vi "Adapt To Type.vi"(7 "Type and Defaults":variant, 8 "error in (no error)":errorcluster, 10 "Variant in":variant, 11 "Deserializer in":refnum<class "JSON Deserializer.lvclass">) -> (0 "error out":errorcluster, 2 "Variant out":variant, 3 "Deserializer out":refnum<class "JSON Deserializer.lvclass">)   [LabVIEW 2017, in "JKI JSON Serialization.lvlib" / "JSON Deserializer.lvclass"]
doc: "Adapts <b>Variant in</b> previously unflattened from a JSON formatted string to match the type of <b>Type and Defaults</b>. For any cluster element in Type and Defaults, the value of the element in Type and Default is used if element with the same name is not present in Variant in."
uses:
  JSON Deserializer.lvclass
  JSON Deserializer.lvclass/JSON Deserializer.ctl
  Library/Waveform Cluster.ctl
  Library/Empty Cluster.vi
  Library/Null Value.vi
  <vilib>/Utility/VariantDataType/VariantType.lvlib
  JKI JSON Serialization.lvlib
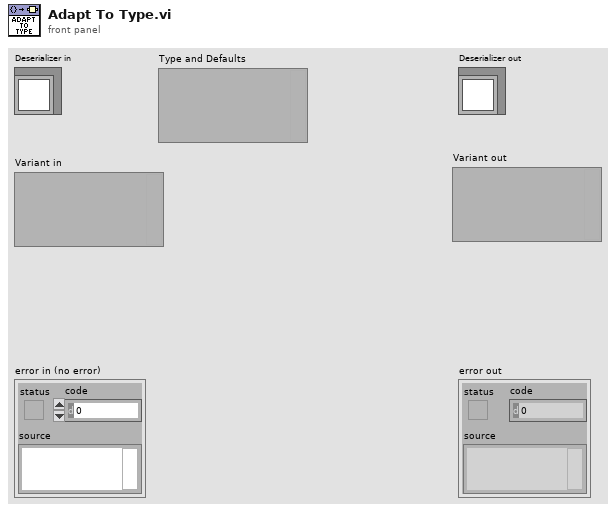
[diagram p1: front panel]
types:
  T1 = typedef "VariantType.lvlib/Type.ctl" = enum8{"Invalid Type", "Void", "I8", "I16", "I32", "I64", "U8", "U16", "U32", "U64", "Single Float", "Double Float", "Extended Float", "Single Complex", "Double Complex", "Extended Complex", "Enum U8", "Enum U16", "Enum U32", "Enum U64", "Single Float With Unit", "Double Float With Unit", "Extended Float With Unit", "Single Complex with Unit", "Double Complex with Unit", "Extended Complex with Unit", "Boolean", "String", "Path", "Picture", "Tag", "Array", "Cluster", "Variant", "LV Variant", "Waveform", "Timestamp", "Digital Waveform", "Digital Data", "ExpressData", "Refnum", "External Data", "VI", "Poly VI", "LabVIEW Class Instance", "Fixed Point"}
  T2 = typedef "JKI JSON Serialization.lvlib/Waveform Cluster.ctl" = cluster{"t0":timestamp, "dt":dbl, "y":dbl[]}
  T3 = typedef "VariantType.lvlib/MemoryInfo.ctl" = cluster{"Type":T4, "Size":u32}
  T4 = typedef "VariantType.lvlib/MemoryType.ctl" = enum16{"Variable", "Fixed", "Bounded"}
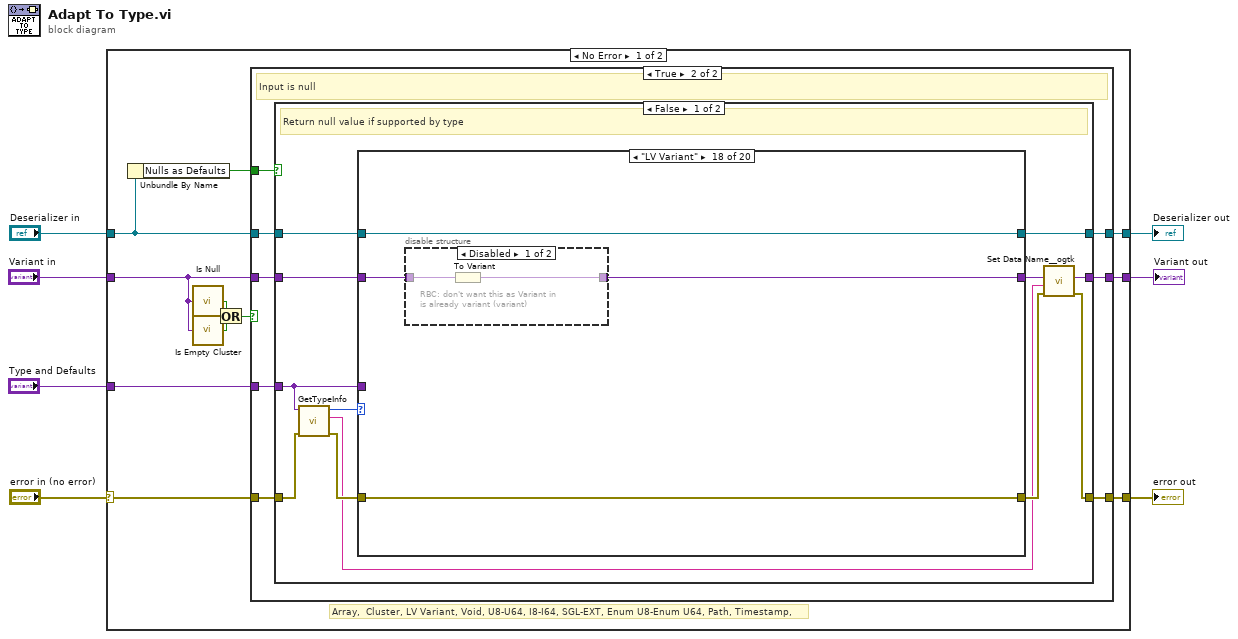
[diagram p0: block diagram]
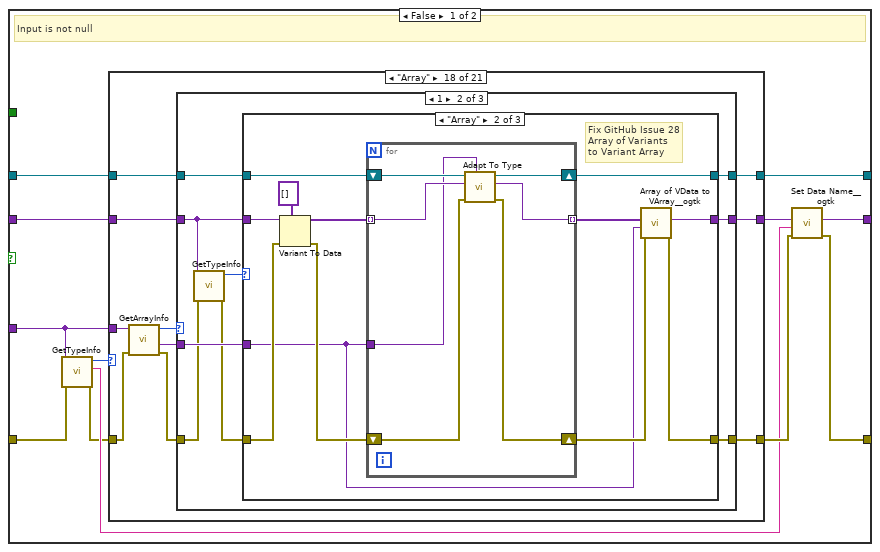
[diagram p2: hidden frame]
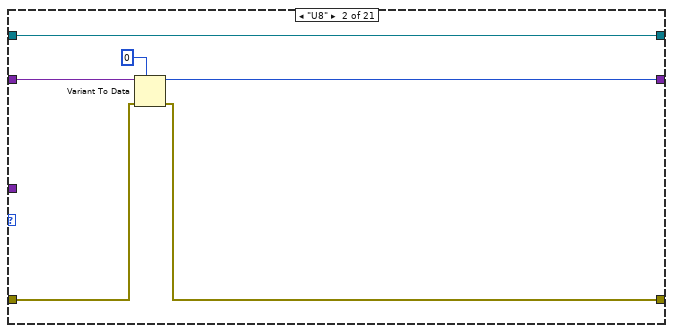
[diagram p4: hidden frame]
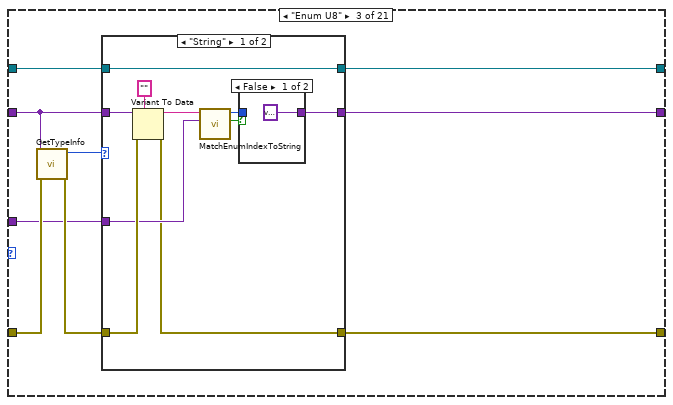
[diagram p5: hidden frame]
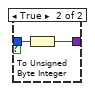
[diagram p6: hidden frame]
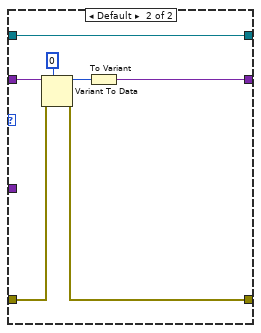
[diagram p7: hidden frame]
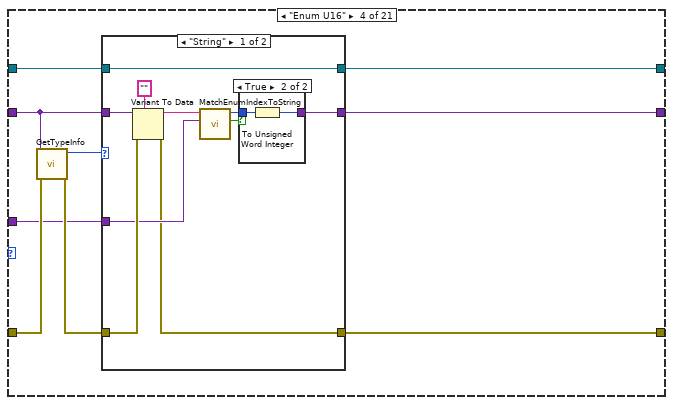
[diagram p8: hidden frame]
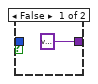
[diagram p9: hidden frame]
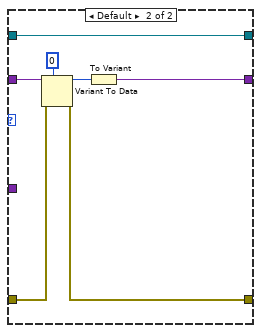
[diagram p10: hidden frame]
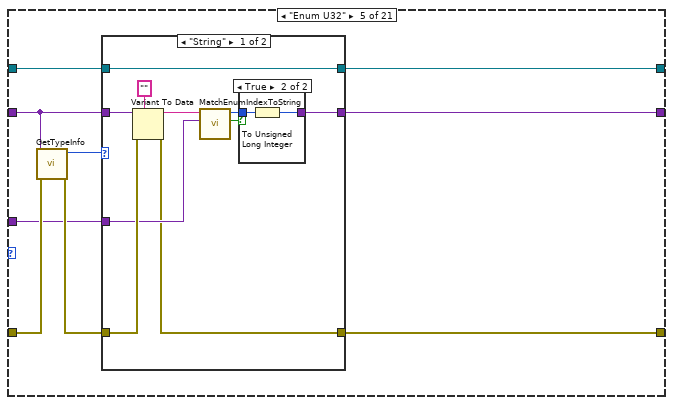
[diagram p11: hidden frame]
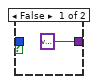
[diagram p12: hidden frame]
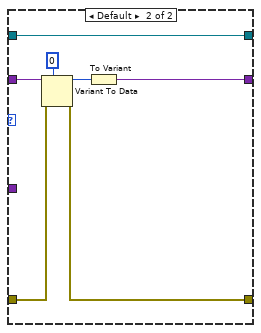
[diagram p13: hidden frame]
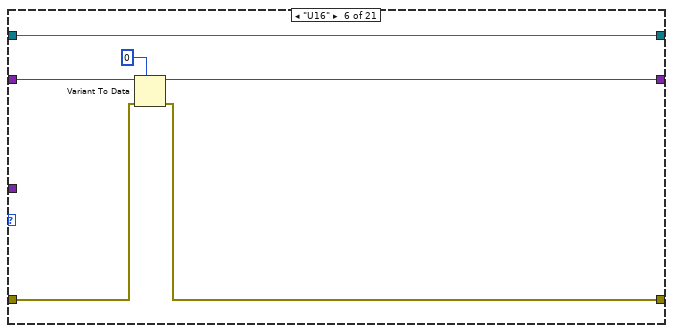
[diagram p14: hidden frame]
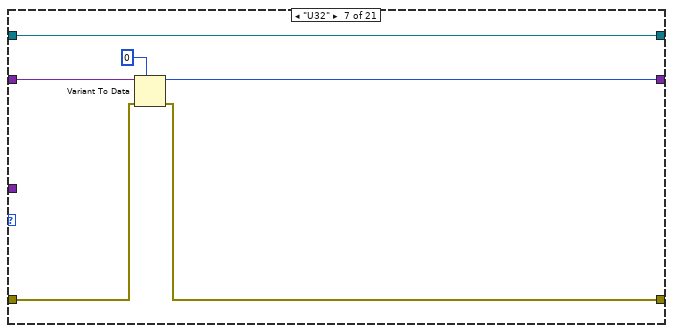
[diagram p15: hidden frame]
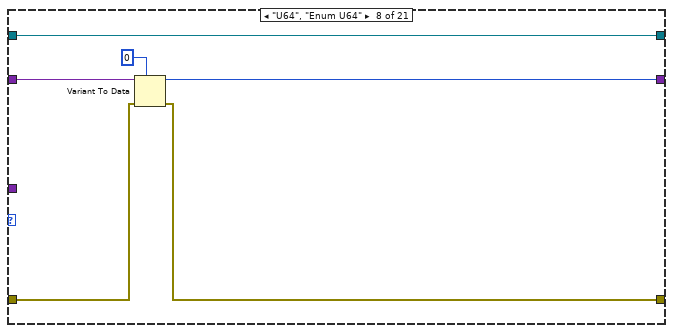
[diagram p16: hidden frame]
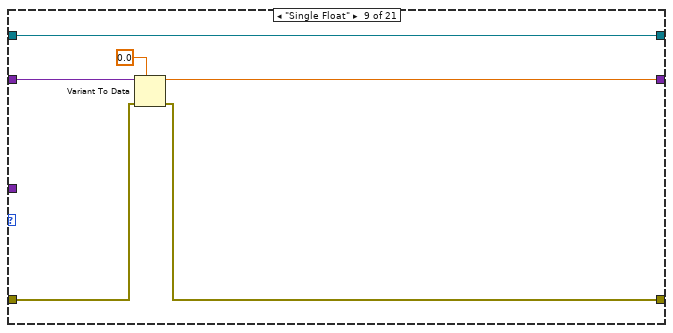
[diagram p17: hidden frame]
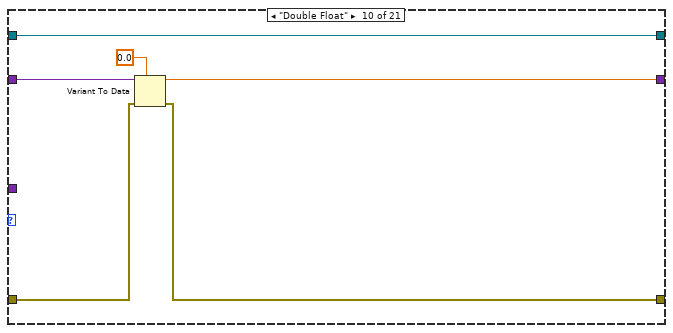
[diagram p18: hidden frame]
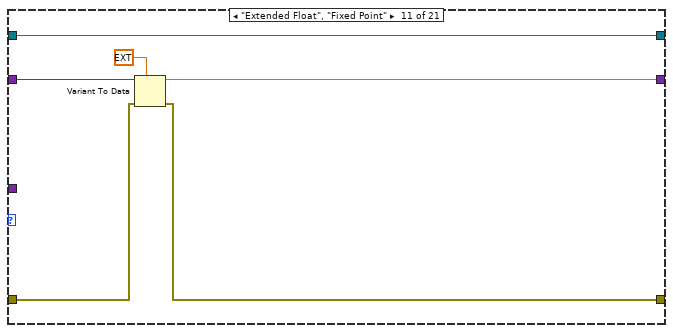
[diagram p19: hidden frame]
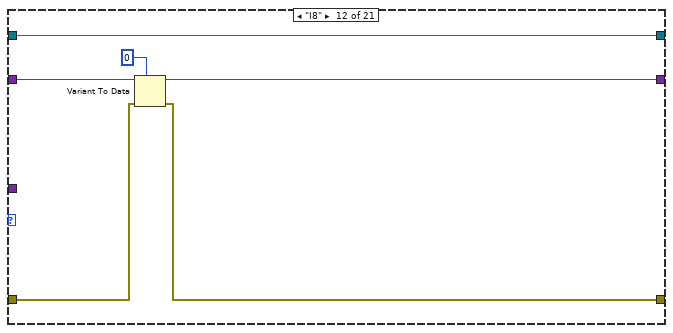
[diagram p20: hidden frame]
diagram:
  n1 = case shown="No Error" "error in (no error)" {
    selector: "error in (no error)" -> [w17 w553]
    tunnel: "Deserializer in" -> [w13 w554]
    tunnel: "Variant in" -> [w11 _]
    tunnel: [w14 w553] -> w4
    tunnel: "Type and Defaults" -> [w16 w552]
    tunnel: [w18 w554] -> w2
    tunnel: [w15 w552] -> w1
    frame No Error {
      # "Array,  Cluster, LV Variant, Void, U8-U64, I8-I64, SGL-EXT, Enum U8-Enum U64, Path, Timestamp,"
      n2 = Unbundle By Name(w13) -> ("Nulls as Defaults"=w12:bool)
      n3 = call "Is Null.vi"("Deserialized JSON Data"=w11) -> ("Null?"=w10:bool)
      n4 = call "Is Empty Cluster.vi"("Deserialized JSON Data"=w11) -> ("Empty Cluster?"=w9:bool)
      n5 = Or(x=w10, y=w9) -> (x .or. y?=w8:bool)
      n6 = case shown="True" w8 {
        tunnel: w13 -> [w20 w434]
        tunnel: [w19 w433] -> w18
        tunnel: w17 -> [w29 w431]
        tunnel: w16 -> [w28 w435]
        tunnel: [w26 w436] -> w15
        tunnel: [w25 w430] -> w14
        tunnel: w11 -> [w21 w432]
        tunnel: w12 -> [_ w429]
        frame False {
          # "Input is not null"
          n7 = call <vilib>:"GetTypeInfo.vi"("error in (no error)"=w29, "Variant"=w28) -> ("error out"=w22:errorcluster, "Name"=w23:string, "Type Enum"=w30:T1)  [unwired: 5 in, 2 out]
          n8 = case shown="\"Array\"" w30 {
            tunnel: [w32 w36 w46 w75 w104 w129 w135 w141 w147 w153 w159 w165 w171 w177 w183 w192 w195 w208 w293 w376 w426] -> w24
            tunnel: w22 -> [w32 w37 w44 w73 w102 w130 w136 w142 w148 w154 w160 w166 w172 w178 w184 w189 w199 w210 w292 w375 w426]
            tunnel: w20 -> [w33 w39 w42 w71 w100 w132 w138 w144 w150 w156 w162 w168 w174 w180 w186 w193 w201 w207 w297 w380 w428]
            tunnel: [w33 w39 w41 w70 w99 w132 w138 w144 w150 w156 w162 w168 w174 w180 w186 w193 w201 w205 w296 w379 w428] -> w19
            tunnel: w28 -> [_ _ w40 w69 w98 _ _ _ _ _ _ _ _ _ _ _ _ w211 w295 w378 _]
            tunnel: w21 -> [w31 w38 w47 w76 w105 w131 w137 w143 w149 w155 w161 w167 w173 w179 w185 w190 w200 w202 w290 w373 w427]
            tunnel: [w31 w34 w48 w77 w106 w127 w133 w139 w145 w151 w157 w163 w169 w175 w181 w191 w194 w204 w294 w377 w425] -> w27
            frame "Void", Default {
            }
            frame "U8" {
              n9 = Variant To Data(error in=w37, type=u8 0, Variant=w38) -> (data=w34:u8, error out=w36:errorcluster)
            }
            frame "Enum U8" {
              n10 = call <vilib>:"GetTypeInfo.vi"("error in (no error)"=w44, "Variant"=w47) -> ("error out"=w43:errorcluster, "Type Enum"=w45:T1)  [unwired: 5 in, 3 out]
              n11 = case shown="\"String\"" w45 {
                tunnel: [w52 w62] -> w48
                tunnel: w47 -> [w58 w66]
                tunnel: w43 -> [w56 w65]
                tunnel: [w49 w64] -> w46
                tunnel: w42 -> [w50 w63]
                tunnel: [w50 w63] -> w41
                tunnel: w40 -> [w54 _]
                frame "String" {
                  n12 = Variant To Data(error in=w56, type="", Variant=w58) -> (data=w55:string, error out=w49:errorcluster)
                  n13 = call "MatchEnumIndexToString.vi"("Enum Variant"=w54, "String"=w55) -> ("found"=w51:bool, "index"=w53:i32)  [unwired: 8 in]
                  n14 = case shown="False" w51 {
                    tunnel: w53 -> [_ w61]
                    tunnel: [variant ("Type and Defaults") w60] -> w52
                    frame False {
                    }
                    frame True {
                      n15 = To Unsigned Byte Integer(number=w61) -> (unsigned 8bit integer=w60:u8)
                    }
                  }
                }
                frame Default {
                  n16 = Variant To Data(error in=w65, type=u8 0, Variant=w66) -> (data=w67:u8, error out=w64:errorcluster)
                  n17 = To Variant(anything=w67) -> (Variant=w62:variant)
                }
              }
            }
            frame "Enum U16" {
              n18 = call <vilib>:"GetTypeInfo.vi"("error in (no error)"=w73, "Variant"=w76) -> ("error out"=w72:errorcluster, "Type Enum"=w74:T1)  [unwired: 5 in, 3 out]
              n19 = case shown="\"String\"" w74 {
                tunnel: [w81 w91] -> w77
                tunnel: w76 -> [w87 w95]
                tunnel: w72 -> [w85 w94]
                tunnel: [w78 w93] -> w75
                tunnel: w71 -> [w79 w92]
                tunnel: [w79 w92] -> w70
                tunnel: w69 -> [w83 _]
                frame "String" {
                  n20 = Variant To Data(error in=w85, type="", Variant=w87) -> (data=w84:string, error out=w78:errorcluster)
                  n21 = call "MatchEnumIndexToString.vi"("Enum Variant"=w83, "String"=w84) -> ("found"=w80:bool, "index"=w82:i32)  [unwired: 8 in]
                  n22 = case shown="True" w80 {
                    tunnel: w82 -> [_ w90]
                    tunnel: [variant ("Type and Defaults") w89] -> w81
                    frame False {
                    }
                    frame True {
                      n23 = To Unsigned Word Integer(number=w90) -> (unsigned 16bit integer=w89:u16)
                    }
                  }
                }
                frame Default {
                  n24 = Variant To Data(error in=w94, type=u16 0, Variant=w95) -> (data=w96:u16, error out=w93:errorcluster)
                  n25 = To Variant(anything=w96) -> (Variant=w91:variant)
                }
              }
            }
            frame "Enum U32" {
              n26 = call <vilib>:"GetTypeInfo.vi"("error in (no error)"=w102, "Variant"=w105) -> ("error out"=w101:errorcluster, "Type Enum"=w103:T1)  [unwired: 5 in, 3 out]
              n27 = case shown="\"String\"" w103 {
                tunnel: [w110 w120] -> w106
                tunnel: w105 -> [w116 w124]
                tunnel: w101 -> [w114 w123]
                tunnel: [w107 w122] -> w104
                tunnel: w100 -> [w108 w121]
                tunnel: [w108 w121] -> w99
                tunnel: w98 -> [w112 _]
                frame "String" {
                  n28 = Variant To Data(error in=w114, type="", Variant=w116) -> (data=w113:string, error out=w107:errorcluster)
                  n29 = call "MatchEnumIndexToString.vi"("Enum Variant"=w112, "String"=w113) -> ("found"=w109:bool, "index"=w111:i32)  [unwired: 8 in]
                  n30 = case shown="True" w109 {
                    tunnel: w111 -> [_ w119]
                    tunnel: [variant ("Type and Defaults") w118] -> w110
                    frame False {
                    }
                    frame True {
                      n31 = To Unsigned Long Integer(number=w119) -> (unsigned 32bit integer=w118:u32)
                    }
                  }
                }
                frame Default {
                  n32 = Variant To Data(error in=w123, type=u32 0, Variant=w124) -> (data=w125:u32, error out=w122:errorcluster)
                  n33 = To Variant(anything=w125) -> (Variant=w120:variant)
                }
              }
            }
            frame "U16" {
              n34 = Variant To Data(error in=w130, type=u16 0, Variant=w131) -> (data=w127:u16, error out=w129:errorcluster)
            }
            frame "U32" {
              n35 = Variant To Data(error in=w136, type=u32 0, Variant=w137) -> (data=w133:u32, error out=w135:errorcluster)
            }
            frame "U64", "Enum U64" {
              n36 = Variant To Data(error in=w142, type=u64 0, Variant=w143) -> (data=w139:u64, error out=w141:errorcluster)
            }
            frame "Single Float" {
              n37 = Variant To Data(error in=w148, type=sgl 0.0, Variant=w149) -> (data=w145:sgl, error out=w147:errorcluster)
            }
            frame "Double Float" {
              n38 = Variant To Data(error in=w154, type=0.0, Variant=w155) -> (data=w151:dbl, error out=w153:errorcluster)
            }
            frame "Extended Float", "Fixed Point" {
              n39 = Variant To Data(error in=w160, type=ext 0.0, Variant=w161) -> (data=w157:ext, error out=w159:errorcluster)
            }
            frame "I8" {
              n40 = Variant To Data(error in=w166, type=i8 0, Variant=w167) -> (data=w163:i8, error out=w165:errorcluster)
            }
            frame "I16" {
              n41 = Variant To Data(error in=w172, type=i16 0, Variant=w173) -> (data=w169:i16, error out=w171:errorcluster)
            }
            frame "I32" {
              n42 = Variant To Data(error in=w178, type=0, Variant=w179) -> (data=w175:i32, error out=w177:errorcluster)
            }
            frame "I64" {
              n43 = Variant To Data(error in=w184, type=i64 0, Variant=w185) -> (data=w181:i64, error out=w183:errorcluster)
            }
            frame "Path" {
              n44 = Variant To Data(error in=w189, type="", Variant=w190) -> (data=w187:string, error out=w192:errorcluster)
              n45 = String To Path(string=w187) -> (path=w191:path)
            }
            frame "Timestamp" {
              n46 = Variant To Data(error in=w199, type="", Variant=w200) -> (data=w197:string, error out=w196:errorcluster)
              n47 = call "ISO String To Timestamp.vi"("error in (no error)"=w196, "ISO Timestamp String"=w197) -> ("error out"=w195:errorcluster, "Time Stamp"=w194:timestamp)  [unwired: 8 in]
            }
            frame "Array" {
              n48 = call <vilib>:"GetArrayInfo.vi"("error in (no error)"=w210, "Variant"=w211) -> ("error out"=w209:errorcluster, "ArrayElement"=w206:variant, "NDims"=w203:i32)  [unwired: 6 in, 1 out]
              n49 = case shown="1" w203 {
                tunnel: w209 -> [w214 w221 w270]
                tunnel: w202 -> [w216 w219 w268]
                tunnel: [w215 w226 w275] -> w208
                tunnel: w207 -> [w217 w225 w274]
                tunnel: w206 -> [_ w224 w273]
                tunnel: [w217 w223 w272] -> w205
                tunnel: [w216 w222 w271] -> w204
                frame 0, Default {
                  n50 = call <vilib>:"Error Cluster From Error Code.vi"("error in (no error)"=w214, "error message (\"\")"="Unflattening failed. Zero dimensional arrays not supported." ("error message (\"\")"), "error code (0)"=1) -> ("error out"=w215:errorcluster)  [unwired: 6 in]
                }
                frame 1 {
                  n51 = call <vilib>:"GetTypeInfo.vi"("error in (no error)"=w221, "Variant"=w219) -> ("error out"=w220:errorcluster, "Type Enum"=w218:T1)  [unwired: 5 in, 3 out]
                  n52 = case shown="\"Array\"" w218 {
                    tunnel: [w227 w232 w249] -> w226
                    tunnel: w225 -> [w229 w238 w259]
                    tunnel: w224 -> [w228 w231 w258]
                    tunnel: [w229 w237 w257] -> w223
                    tunnel: [w228 w234 w251] -> w222
                    tunnel: w220 -> [w227 w236 w254]
                    tunnel: w219 -> [_ w235 w256]
                    frame Default {
                    }
                    frame "Array" {
                      # "Fix GitHub Issue 28\nArray of Variants\nto Variant Array"
                      n53 = Variant To Data(error in=w236, type=variant[] [], Variant=w235) -> (data=w240:variant[], error out=w239:errorcluster)
                      n54 = for {
                        tunnel: w240 -> [w247] mode=indexing
                        shift-right: [w245] -> w233
                        shift-left: w239 -> [w246]
                        shift-right: [w243] -> w237
                        shift-left: w238 -> [w248]
                        tunnel: w231 -> [w244]
                        tunnel: [w242] -> w230 mode=indexing
                        n55 = call-dynamic "Adapt To Type.vi"("Type and Defaults"=w244, "error in (no error)"=w246, "Variant in"=w247, "Deserializer in"=w248) -> ("error out"=w245:errorcluster, "Variant out"=w242:variant, "Deserializer out"=w243:refnum<class "JSON Deserializer.lvclass">)  [unwired: 5 in]
                      }
                      n56 = call <userlib>:"Array of VData to VArray__ogtk.vi"("error in (no error)"=w233, "Element Type (when empty)"=w231, "1D Array of VData"=w230) -> ("error out"=w232:errorcluster, "VArray"=w234:variant)  [unwired: 7 in]
                    }
                    frame "Cluster" {
                      # "Fix GitHub Issue 29\nArray of Variants\nto Variant Cluster"
                      n57 = call <userlib>:"Cluster to Array of VData__ogtk.vi"("error in (no error)"=w254, "Cluster"=w256) -> ("error out"=w255:errorcluster, "Array of VData"=w253:variant[])  [unwired: 8 in]
                      n58 = for {
                        tunnel: w253 -> [w265] mode=indexing
                        shift-right: [w263] -> w250
                        shift-left: w255 -> [w264]
                        shift-right: [w261] -> w257
                        shift-left: w259 -> [w266]
                        tunnel: w258 -> [w262]
                        tunnel: [w260] -> w252 mode=indexing
                        n59 = call-dynamic "Adapt To Type.vi"("Type and Defaults"=w262, "error in (no error)"=w264, "Variant in"=w265, "Deserializer in"=w266) -> ("error out"=w263:errorcluster, "Variant out"=w260:variant, "Deserializer out"=w261:refnum<class "JSON Deserializer.lvclass">)  [unwired: 5 in]
                      }
                      n60 = call <userlib>:"Array of VData to VCluster__ogtk.vi"("error in (no error)"=w250, "Array"=w252) -> ("error out"=w249:errorcluster, "VCluster"=w251:variant)  [unwired: 8 in]
                    }
                  }
                }
                frame 2.. {
                  n61 = call <vilib>:"GetTypeInfo.vi"("error in (no error)"=w270, "Variant"=w268) -> ("error out"=w269:errorcluster, "Type Enum"=w267:T1)  [unwired: 5 in, 3 out]
                  n62 = case shown="\"Array\"" w267 {
                    tunnel: [w276 w283] -> w275
                    tunnel: w274 -> [w278 w280]
                    tunnel: w273 -> [w277 w281]
                    tunnel: [w278 w279] -> w272
                    tunnel: [w277 w282] -> w271
                    tunnel: w269 -> [w276 w287]
                    tunnel: w268 -> [_ w286]
                    frame Default {
                    }
                    frame "Array" {
                      n63 = Variant To Data(error in=w287, type=variant[] [], Variant=w286) -> (data=w285:variant[], error out=w284:errorcluster)
                      n64 = call "Hierarchical VArray to MultiD Array.vi"("error in (no error)"=w284, "Element Type"=w281, "Hierarchical Array"=w285, "Deserializer in"=w280) -> ("error out"=w283:errorcluster, "MultiD Array"=w282:variant, "Deserializer out"=w279:refnum<class "JSON Deserializer.lvclass">)  [unwired: 5 in]
                    }
                  }
                }
              }
            }
            frame "Cluster" {
              n65 = call <vilib>:"GetTypeInfo.vi"("error in (no error)"=w292, "Variant"=w290) -> ("error out"=w291:errorcluster, "Type Enum"=w289:T1)  [unwired: 5 in, 3 out]
              n66 = case shown="\"Cluster\"" w289 {
                tunnel: w297 -> [w303 w306 w312 w344]
                tunnel: [w303 w306 w311 w343] -> w296
                tunnel: w295 -> [w302 w305 w318 w342]
                tunnel: [w302 w305 w309 w334] -> w294
                tunnel: [w301 w304 w307 w331] -> w293
                tunnel: w291 -> [w300 w304 w317 w330]
                tunnel: w290 -> [_ _ w319 w329]
                frame "Invalid Type", Default {
                  n67 = call <vilib>:"Error Cluster From Error Code.vi"("error in (no error)"=w300, "error message (\"\")"="Cannot deserialize the input type into a cluster." ("error message (\"\")"), "error code (0)"=1) -> ("error out"=w301:errorcluster)  [unwired: 6 in]
                }
                frame "Void" {
                  # "Empty input object, use default values"
                }
                frame "Array" {
                  n68 = call <userlib>:"Cluster to Array of VData__ogtk.vi"("error in (no error)"=w317, "Cluster"=w318) -> ("error out"=w316:errorcluster, "Array of VData"=w315:variant[])  [unwired: 8 in]
                  n69 = call <userlib>:"Array to Array of VData__ogtk.vi"("error in (no error)"=w316, "MultiD Array"=w319) -> ("error out"=w313:errorcluster, "1D Array of Variants"=w314:variant[])  [unwired: 8 in]
                  n70 = for {
                    tunnel: w315 -> [w324] mode=indexing
                    tunnel: w314 -> [w327]
                    shift-right: [w322] -> w308
                    shift-left: w313 -> [w323]
                    shift-right: [w321] -> w311
                    shift-left: w312 -> [w328]
                    tunnel: [w320] -> w310 mode=indexing
                    i -> [w326]
                    n71 = Index Array(array=w327, index=w326) -> (element=w325:variant)
                    n72 = call-dynamic "Adapt To Type.vi"("Type and Defaults"=w324, "error in (no error)"=w323, "Variant in"=w325, "Deserializer in"=w328) -> ("error out"=w322:errorcluster, "Variant out"=w320:variant, "Deserializer out"=w321:refnum<class "JSON Deserializer.lvclass">)  [unwired: 5 in]
                  }
                  n73 = call <userlib>:"Array of VData to VCluster__ogtk.vi"("error in (no error)"=w308, "Array"=w310) -> ("error out"=w307:errorcluster, "VCluster"=w309:variant)  [unwired: 8 in]
                }
                frame "Cluster" {
                  n74 = call <userlib>:"Cluster to Array of VData__ogtk.vi"("error in (no error)"=w330, "Cluster"=w342) -> ("error out"=w340:errorcluster, "Array of VData"=w341:variant[])  [unwired: 8 in]
                  n75 = call <userlib>:"Cluster to Array of VData__ogtk.vi"("error in (no error)"=w340, "Cluster"=w329) -> ("error out"=w336:errorcluster, "Array of VData"=w339:variant[])  [unwired: 8 in]
                  n76 = for {
                    tunnel: w339 -> [w346] mode=indexing
                    shift-right: [w347] -> w335
                    shift-left: w336 -> [w348]
                    tunnel: [w346] -> w338 mode=indexing
                    tunnel: [w345] -> w337 mode=indexing
                    n77 = call <vilib>:"GetTypeInfo.vi"("error in (no error)"=w348, "Variant"=w346) -> ("error out"=w347:errorcluster, "Name"=w345:string)  [unwired: 5 in, 3 out]
                  }
                  n78 = for {
                    shift-right: [w358] -> w332
                    shift-left: w335 -> [w353]
                    shift-right: [w357] -> w343
                    shift-left: w344 -> [w359]
                    tunnel: w341 -> [w350] mode=indexing
                    tunnel: [w356] -> w333 mode=indexing
                    tunnel: w338 -> [w351]
                    tunnel: w337 -> [w355]
                    n79 = call <vilib>:"GetTypeInfo.vi"("error in (no error)"=w353, "Variant"=w350) -> ("error out"=w352:errorcluster, "Name"=w354:string)  [unwired: 5 in, 3 out]
                    n80 = Search 1D Array(1D array=w355, element=w354) -> (index of element=w349:i32)  [unwired: 1 in]
                    n81 = case shown="0.." w349 {
                      selector: w349 -> [_ w363]
                      tunnel: w359 -> [w362 w371]
                      tunnel: [w360 w370] -> w358
                      tunnel: [w362 w369] -> w357
                      tunnel: [w361 w368] -> w356
                      tunnel: w352 -> [w360 w367]
                      tunnel: w351 -> [_ w366]
                      tunnel: w350 -> [w361 w364]
                      frame ..-1 {
                        # "Element not found"
                      }
                      frame 0.. {
                        # "Element found"
                        n82 = Index Array(array=w366, index=w363) -> (element=w365:variant)
                        n83 = call-dynamic "Adapt To Type.vi"("Type and Defaults"=w364, "error in (no error)"=w367, "Variant in"=w365, "Deserializer in"=w371) -> ("error out"=w370:errorcluster, "Variant out"=w368:variant, "Deserializer out"=w369:refnum<class "JSON Deserializer.lvclass">)  [unwired: 5 in]
                      }
                    }
                  }
                  n84 = call <userlib>:"Array of VData to VCluster__ogtk.vi"("error in (no error)"=w332, "Array"=w333) -> ("error out"=w331:errorcluster, "VCluster"=w334:variant)  [unwired: 8 in]
                }
              }
            }
            frame "Waveform" {
              n85 = call <vilib>:"GetTypeInfo.vi"("error in (no error)"=w375, "Variant"=w373) -> ("error out"=w374:errorcluster, "Type Enum"=w372:T1)  [unwired: 5 in, 3 out]
              n86 = case shown="\"Array\"" w372 {
                tunnel: w380 -> [w386 w389 w404 w421]
                tunnel: [w386 w389 w391 w414] -> w379
                tunnel: w378 -> [w385 w388 w406 w423]
                tunnel: [w385 w388 w390 w413] -> w377
                tunnel: [w384 w387 w392 w415] -> w376
                tunnel: w374 -> [w383 w387 w405 w422]
                tunnel: w373 -> [_ _ w402 w420]
                frame "Invalid Type", Default {
                  n87 = call <vilib>:"Error Cluster From Error Code.vi"("error in (no error)"=w383, "error message (\"\")"="Cannot deserialize the input type into a waveform." ("error message (\"\")"), "error code (0)"=1) -> ("error out"=w384:errorcluster)  [unwired: 6 in]
                }
                frame "Void" {
                  # "Empty input object, use default values"
                }
                frame "Cluster" {
                  w398 = T2 {"t0"=timestamp(0 s since 1904-01-01), "dt"=1.0, "y"=[]}  # waveform
                  n88 = Variant To Data(error in=w405, type=waveform(dbl) {"t0"=timestamp(0 s since 1904-01-01), "dt"=1.0, "Y"=[]}, Variant=w406) -> (data=w397:waveform(dbl), error out=w401:errorcluster)
                  n89 = Unbundle By Name(w397) -> ("t0"=w409:timestamp, "dt"=w408:dbl, "Y"=w407:dbl[])
                  n90 = Bundle By Name(cluster=w398, "t0"=w409, "dt"=w408, "y"=w407) -> (w403:T2)
                  n91 = call-dynamic "Adapt To Type.vi"("Type and Defaults"=w403, "error in (no error)"=w401, "Variant in"=w402, "Deserializer in"=w404) -> ("error out"=w399:errorcluster, "Variant out"=w400:variant, "Deserializer out"=w391:refnum<class "JSON Deserializer.lvclass">)  [unwired: 5 in]
                  n92 = Variant To Data(error in=w399, type=w398, Variant=w400) -> (data=w396:T2, error out=w392:errorcluster)
                  n93 = Unbundle By Name(w396) -> ("t0"=w395:timestamp, "dt"=w394:dbl, "y"=w393:dbl[])
                  n94 = Bundle By Name(cluster=w397, "t0"=w395, "dt"=w394, "Y"=w393) -> (w390:waveform(dbl))
                }
                frame "Array" {
                  n95 = Variant To Data(error in=w422, type=waveform(dbl) {"t0"=timestamp(0 s since 1904-01-01), "dt"=1.0, "Y"=[]}, Variant=w423) -> (data=w416:waveform(dbl), error out=w419:errorcluster)
                  n96 = Unbundle By Name(w416) -> ("Y"=w412:dbl[])
                  n97 = call-dynamic "Adapt To Type.vi"("Type and Defaults"=w412, "error in (no error)"=w419, "Variant in"=w420, "Deserializer in"=w421) -> ("error out"=w417:errorcluster, "Variant out"=w418:variant, "Deserializer out"=w414:refnum<class "JSON Deserializer.lvclass">)  [unwired: 5 in]
                  n98 = Variant To Data(error in=w417, type=w412, Variant=w418) -> (data=w411:dbl[], error out=w415:errorcluster)
                  n99 = Bundle By Name(cluster=w416, "Y"=w411) -> (w413:waveform(dbl))
                }
              }
            }
            frame "LV Variant" {
              n100 = To Variant(anything=w427) -> (Variant=w425:variant)
            }
          }
          n101 = call <userlib>:"Set Data Name__ogtk.vi"("error in (no error)"=w24, "Data Name"=w23, "Data"=w27) -> ("error out"=w25:errorcluster, "Renamed Data"=w26:variant)  [unwired: 7 in]
        }
        frame True {
          # "Input is null"
          n102 = case shown="False" w429 {
            tunnel: [w444 w551] -> w436
            tunnel: w435 -> [w441 w551]
            tunnel: w434 -> [w448 w550]
            tunnel: [w447 w550] -> w433
            tunnel: w432 -> [w446 _]
            tunnel: w431 -> [w440 w549]
            tunnel: [w442 w549] -> w430
            frame False {
              # "Return null value if supported by type"
              n103 = call <vilib>:"GetTypeInfo.vi"("error in (no error)"=w440, "Variant"=w441) -> ("error out"=w439:errorcluster, "Name"=w437:string, "Type Enum"=w438:T1)  [unwired: 5 in, 2 out]
              n104 = case shown="\"LV Variant\"" w438 {
                tunnel: [w450 w452 w455 w458 w461 w464 w467 w470 w473 w476 w479 w482 w485 w488 w491 w494 w497 w502 w509 w521] -> w443
                tunnel: w439 -> [w450 w452 w455 w458 w461 w464 w467 w470 w473 w476 w479 w482 w485 w488 w491 w494 w497 w502 w512 w523]
                tunnel: w448 -> [w451 w454 w457 w460 w463 w466 w469 w472 w475 w478 w481 w484 w487 w490 w493 w496 w499 w503 w513 w520]
                tunnel: [w451 w454 w457 w460 w463 w466 w469 w472 w475 w478 w481 w484 w487 w490 w493 w496 w499 w503 w513 w518] -> w447
                tunnel: w441 -> [_ _ _ _ _ _ _ _ _ _ _ _ _ _ _ _ _ _ w508 w524]
                tunnel: w446 -> [w449 _ _ _ _ _ _ _ _ _ _ _ _ _ _ _ _ w501 _ w515]
                tunnel: [w449 "" path "" waveform(dbl) {"t0"=timestamp(0 s since 1904-01-01), "dt"=1.0, "Y"=[]} FALSE timestamp(0 s since 1904-01-01) sgl nan nan ext nan u8 0 u16 0 u32 0 u64 0 i8 0 i16 0 0 i64 0 w500 w507 w517] -> w445
                frame "Void", Default {
                }
                frame "String" {
                }
                frame "Path" {
                }
                frame "Waveform" {
                }
                frame "Boolean" {
                }
                frame "Timestamp" {
                }
                frame "Single Float" {
                }
                frame "Double Float" {
                }
                frame "Extended Float", "Fixed Point" {
                }
                frame "U8", "Enum U8" {
                }
                frame "U16", "Enum U16" {
                }
                frame "U32", "Enum U32" {
                }
                frame "U64", "Enum U64" {
                }
                frame "I8" {
                }
                frame "I16" {
                }
                frame "I32" {
                }
                frame "I64" {
                }
                frame "LV Variant" {
                  n105 = disable-structure shown="Disabled" {
                    disable-tunnel: w501 -> [w505 w506]
                    disable-tunnel: [w504 w506] -> w500
                    frame Disabled {
                      # "RBC: don't want this as Variant in\nis already variant (variant)"
                      n106 = To Variant(anything=w505) -> (Variant=w504:variant)
                    }
                    frame Enabled {
                    }
                  }
                }
                frame "Cluster" {
                  # "Get cluster default value"
                  n107 = call <vilib>:"GetClusterInfo.vi"("error in (no error)"=w512, "Variant"=w508) -> ("error out"=w510:errorcluster, "Cluster Elements"=w511:variant[])  [unwired: 8 in]
                  n108 = call <vilib>:"SetClusterInfo.vi"("error in (no error)"=w510, "Cluster Elements"=w511, "Variant"=w508) -> ("error out"=w509:errorcluster, "Variant Out"=w507:variant)  [unwired: 7 in]
                }
                frame "Array" {
                  n109 = call <vilib>:"GetArrayInfo.vi"("error in (no error)"=w523, "Variant"=w524) -> ("error out"=w522:errorcluster, "ArrayElement"=w519:variant, "Array Lengths"=w514:T3[], "NDims"=w516:i32)  [unwired: 6 in]
                  n110 = case shown="0, Default" w516 {
                    tunnel: w522 -> [w527 w534 w547]
                    tunnel: w515 -> [w529 _ _]
                    tunnel: [w528 w531 w541] -> w521
                    tunnel: w520 -> [w530 w535 w548]
                    tunnel: w519 -> [_ w533 w546]
                    tunnel: [w530 w535 w548] -> w518
                    tunnel: [w529 w536 w543] -> w517
                    tunnel: w514 -> [_ _ w540]
                    frame 0, Default {
                      n111 = call <vilib>:"Error Cluster From Error Code.vi"("error in (no error)"=w527, "error message (\"\")"="Unflattening failed. Zero dimensional arrays not supported." ("error message (\"\")"), "error code (0)"=1) -> ("error out"=w528:errorcluster)  [unwired: 6 in]
                    }
                    frame 1 {
                      n112 = call <userlib>:"Array of VData to VArray__ogtk.vi"("error in (no error)"=w534, "Element Type (when empty)"=w533, "1D Array of VData"=variant[] []) -> ("error out"=w531:errorcluster, "VArray"=w536:variant)  [unwired: 7 in]
                    }
                    frame 2.. {
                      n113 = Array Size(array=w540) -> (size(s)=w539:i32)
                      n114 = Initialize Array(0, w539) -> (w537:i32[])
                      n115 = call <userlib>:"Array of VData to VArray__ogtk.vi"("error in (no error)"=w547, "Element Type (when empty)"=w546, "1D Array of VData"=variant[] []) -> ("error out"=w542:errorcluster, "VArray"=w544:variant)  [unwired: 7 in]
                      n116 = call <userlib>:"Reshape 1D Array__ogtk.vi"("error in (no error)"=w542, "Size(s)"=w537, "1D Array"=w544) -> ("error out"=w541:errorcluster, "Reshaped VArray"=w543:variant)  [unwired: 7 in]
                    }
                  }
                }
              }
              n117 = call <userlib>:"Set Data Name__ogtk.vi"("error in (no error)"=w443, "Data Name"=w437, "Data"=w445) -> ("error out"=w442:errorcluster, "Renamed Data"=w444:variant)  [unwired: 7 in]
            }
            frame True {
              # "Return default value"
            }
          }
        }
      }
    }
    frame Error {
    }
  }
  "error out" <- w4
  "Deserializer out" <- w2
  "Variant out" <- w1
